vi "updateEnemy.vi"(8 "error in (no error)":errorcluster, 10 "old Enemy":refnum<class "Enemy.lvclass">, 11 "Enemy in":refnum<class "Enemy.lvclass">) -> (0 "error out":errorcluster, 3 "Enemy out":refnum<class "Enemy.lvclass">)   [LabVIEW 2023, in "Enemy.lvclass"]
uses:
  Enemy.lvclass
  Team_class/Team.lvclass/Team.ctl
  Team_class/Read RobotRef.vi
  Team_class/Write RobotRef.vi
  Robot_class/Robot.lvclass
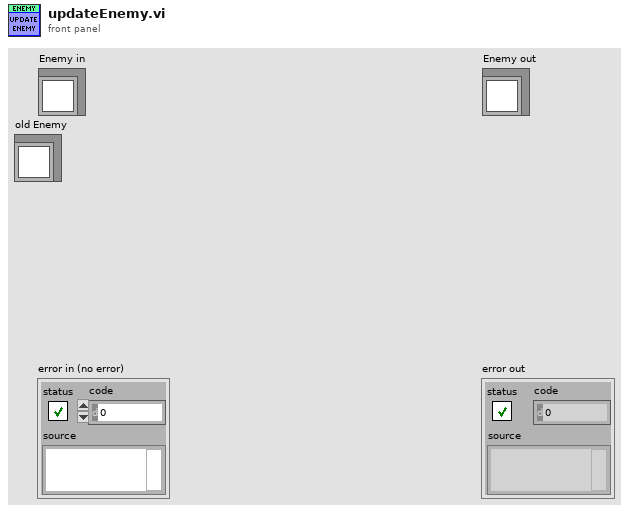
[diagram p1: front panel]
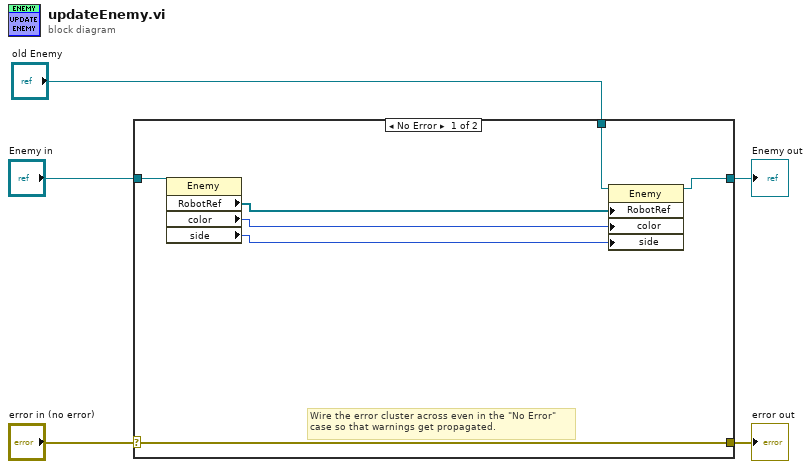
[diagram p0: block diagram]
diagram:
  n1 = case shown="No Error" "error in (no error)" {
    selector: "error in (no error)" -> [w12 w14]
    tunnel: [w12 w14] -> w4
    tunnel: [w10 w13] -> w2
    tunnel: "Enemy in" -> [w11 w13]
    tunnel: "old Enemy" -> [w9 _]
    frame No Error {
      # "Wire the error cluster across even in the \"No Error\"\ncase so that warnings get propagated."
      n2 = property class="Enemy"(reference=w11) -> ("RobotRef"=w8:refnum<class "Robot.lvclass">[], "color"=w7:enum16{"Azul", "Amarelo"}, "side"=w6:enum16{"Esquerdo", "Direito"})  [unwired: 1 in, 2 out]
      n3 = property class="Enemy"(reference=w9, "RobotRef"=w8, "color"=w7, "side"=w6) -> (reference out=w10:refnum<class "Enemy.lvclass">)  [unwired: 1 in, 1 out]
    }
    frame Error {
    }
  }
  "error out" <- w4
  "Enemy out" <- w2
